vi "check_instrument_error.vi"(6 "Mode (Check error from Session)":T1(ring)=enum."Check error from Session", 7 "Attribute":T2={"Identifier"="", "Descriptive Name"="", "Data Type"=enum."Integer 32", "Command"="", "Access"=enum."Read/Write", "Range Table"="", "Read Callback"="", "Write Callback"="", "Supported Models"="", "Instrument Options"="", "Index"=0, "OPC Wait"=FALSE, "No Status Check"=FALSE, "Cache Only"=FALSE}, 8 "error in":errorcluster caption="error in (no error)", 11 "VISA resource name":refnum<visa-resource-name>) -> (0 "error out":errorcluster, 3 "VISA resource name out":refnum<visa-resource-name>)   [LabVIEW 2020, in "Rohde&Schwarz RTx Oscilloscopes.lvlib" / "rsidr_core.lvlib"]
uses:
  rsidr_core.lvlib
  type_Attribute.ctl
  type_Attribute_Data_Type.ctl
  type_ReadWriteAccess.ctl
  type_AdditionalFlag_Bits.ctl
  type_Error_Codes.ctl
  Match Regular Expression.xnode
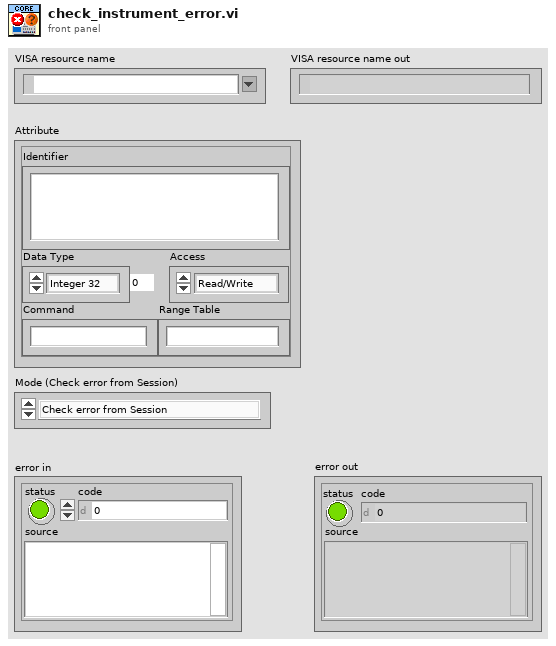
[diagram p1: front panel]
types:
  T1 = enum16{"Check error", "Don't check error", "Check error from Session"}
  T2 = typedef "Rohde&Schwarz RTx Oscilloscopes.lvlib/rsidr_core.lvlib/type_Attribute.ctl" = cluster{"Identifier":string, "Descriptive Name":string, "Data Type":T3, "Command":string, "Access":T4, "Range Table":string, "Read Callback":string, "Write Callback":string, "Supported Models":string, "Instrument Options":string, "Index":i32, "OPC Wait":bool, "No Status Check":bool, "Cache Only":bool}
  T3 = typedef "Rohde&Schwarz RTx Oscilloscopes.lvlib/rsidr_core.lvlib/type_Attribute_Data_Type.ctl" = enum16{"Integer 32", "Double", "String", "Boolean", "None", "Integer 64", "RawString"}
  T4 = typedef "Rohde&Schwarz RTx Oscilloscopes.lvlib/rsidr_core.lvlib/type_ReadWriteAccess.ctl" = enum16{"Read Only", "Write Only", "Read/Write"}
  T5 = typedef "Rohde&Schwarz RTx Oscilloscopes.lvlib/rsidr_core.lvlib/type_AdditionalFlag_Bits.ctl" = enum16{"Send LF after Bin Block", "Junk read with io_clear_buffers.vi", "io_clear_buffers: viClear()", "io_clear_buffers: viFlush()", "<NotUsed1>", "Allow Dbl & Int Bin/Ascii read", "*OPC? in check_instrument_error.vi", "<NotUsed2>", "Smart Enum Matching", "Less Strict RepCaps check", "AssureResponseEndWithLF"}
  T6 = typedef "Rohde&Schwarz RTx Oscilloscopes.lvlib/rsidr_core.lvlib/type_Session_Data.ctl" = cluster{"IDN string":string, "Instrument FW":string, "Instr type":string, "Instr type for err. msg.":string, "Installed Options":string[], "Ignore Error Messages":string, "Logging params":variant, "OPC Timeout":i32, "VISA Timeout":i32, "STB Poll VISA Timeout":i32, "Additional Flags":i32, "Wait Before Read":i32, "Wait Before Write":i32, "Option String Flags":i32, "IO Segment Size":i64, "VISA Access Mode":T7, "Interface Type":T8, "OPC Wait Mode":T9, "Bin Float Number  Format":T10, "Bin Integer Number Format":T11, "Simulate":bool, "VXIcapable":bool, "Duplicate Session":bool, "Add LF to Write":bool, "Logging":bool, "Fast Sweep":bool, "Query Instrument Status":bool, "Check Range":bool, "Check Options":bool, "OPC-sync Attr Writes":bool, "OPC-sync Attr Queries":bool}
  T7 = typedef "Rohde&Schwarz RTx Oscilloscopes.lvlib/rsidr_core.lvlib/type_VisaAccessMode.ctl" = u16
  T8 = typedef "Rohde&Schwarz RTx Oscilloscopes.lvlib/rsidr_core.lvlib/type_InterfaceType.ctl" = enum16{"Unknown", "GPIB", "VXI", "GPIB_VXI", "ASRL", "PXI", "TCPIP", "USB", "SOCKET"}
  T9 = typedef "Rohde&Schwarz RTx Oscilloscopes.lvlib/rsidr_core.lvlib/type_OPC_Wait_Mode.ctl" = enum16{"STBpolling", "STBpollingSlow", "STBpollingSuperSlow", "ServiceRequest", "OPCquery"}
  T10 = typedef "Rohde&Schwarz RTx Oscilloscopes.lvlib/rsidr_core.lvlib/type_Binary_Float_Number_Format.ctl" = enum16{"Float_4_Bytes_Swapped", "Float_4_Bytes", "Double_8_Bytes_Swapped", "Double_8_Bytes"}
  T11 = typedef "Rohde&Schwarz RTx Oscilloscopes.lvlib/rsidr_core.lvlib/type_Binary_Integer_Number_Format.ctl" = enum16{"Int32_4_Bytes_Swapped", "Int32_4 Bytes", "Int16_2_Bytes_Swapped", "Int16_2_Bytes"}
  T12 = typedef "Rohde&Schwarz RTx Oscilloscopes.lvlib/rsidr_core.lvlib/type_Error_Codes.ctl" = enum16{"No_error", "VISA_err_ResourceNotFound", "VISA_err_Timeout", "VISA_warn_MoreDataAvailable", "RS_err_MissingCallback", "RS_err_InvalidAttribute", "RS_err_InvalidValue", "RS_err_UnknownResource", "RS_err_AlreadyInitialized", "RS_err_InstrumentStatus", "RS_err_BadRepCapName", "RS_err_TypesMismatch", "RS_err_ValueNotSupported", "RS_err_InvalidRngTable", "RS_err_IDqueryFail", "RS_err_UnexpResponse", "VISA_warn_ConfigNotLoaded", "RS_err_AttributeNotReadable", "RS_err_AttributeNotWritable", "RS_err_InstrumentType", "RS_err_InstrumentOption", "VISA_err_InvalidSize", "RS_err_ReliabilityIndicator", "VISA_warn_UnknownStatus", "VISA_warn_TermCharRead", "VISA_err_IO_error", "RS_err_FunctionNotSupported", "VISA_warn_QueueEmpty"}
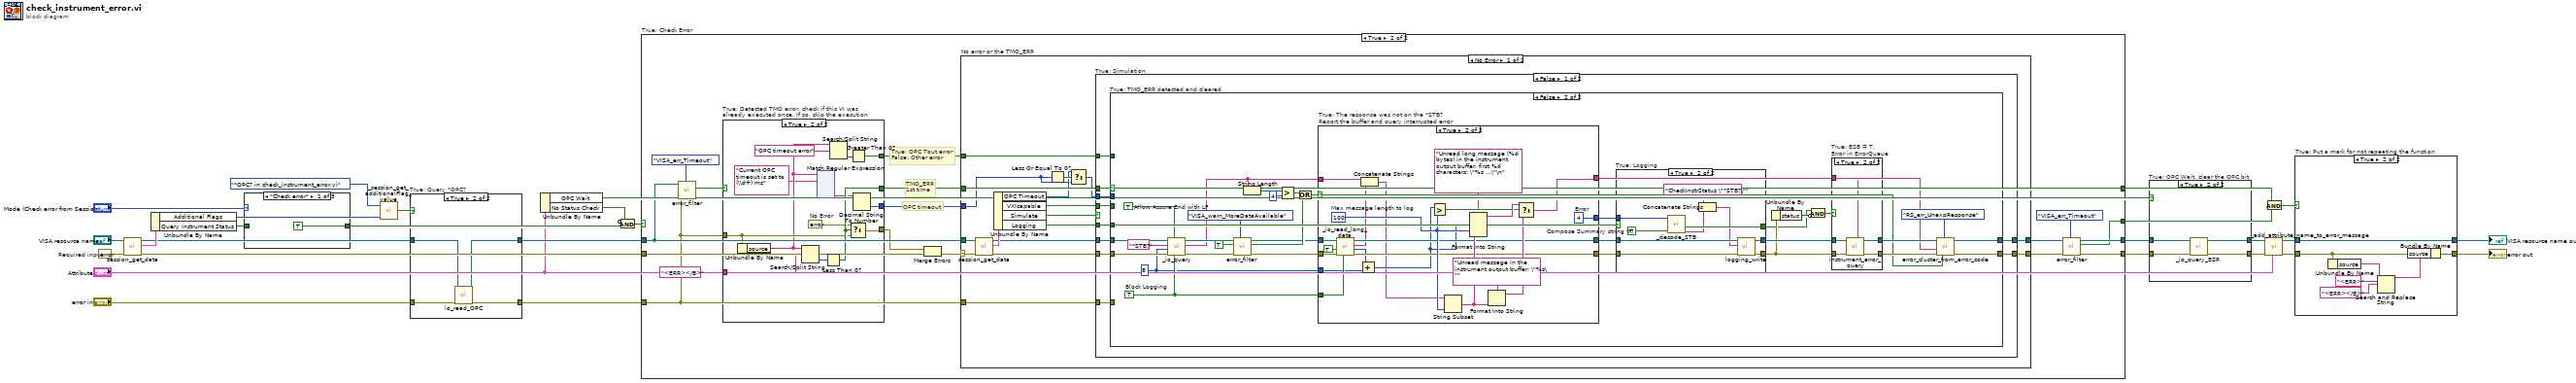
[diagram p0: block diagram]
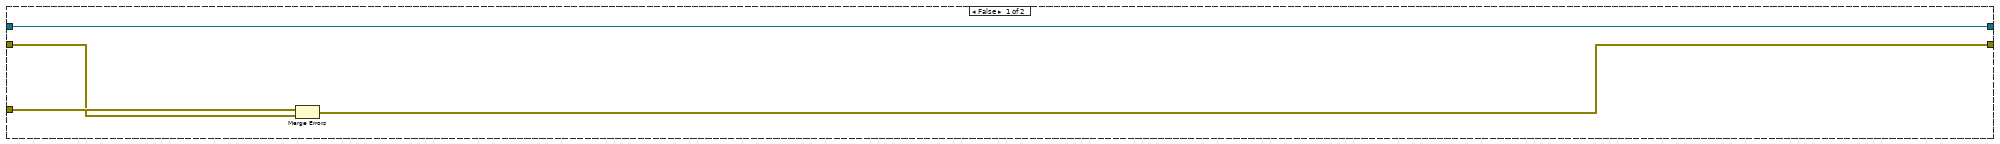
[diagram p5: hidden frame]
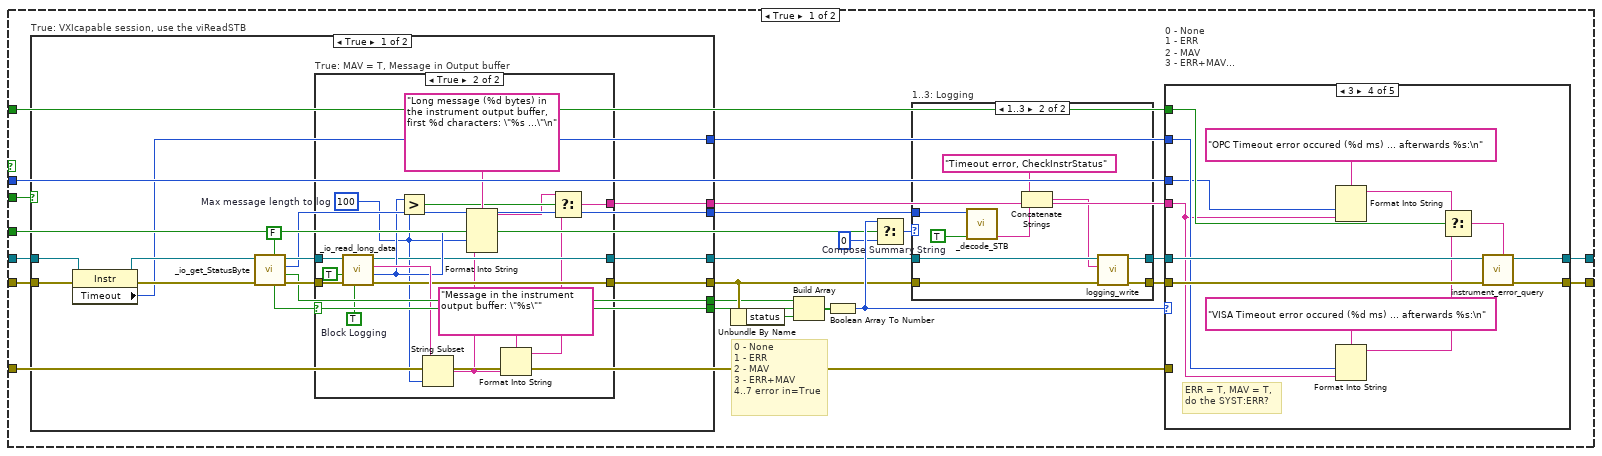
[diagram p7: hidden frame]
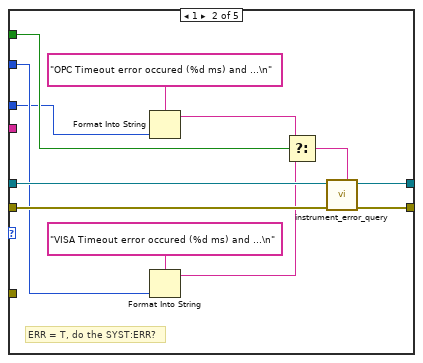
[diagram p9: hidden frame]
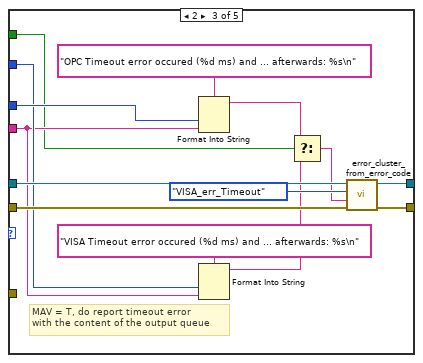
[diagram p10: hidden frame]
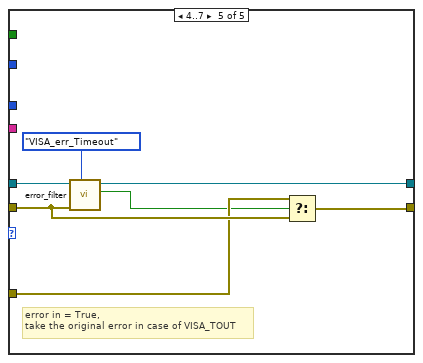
[diagram p11: hidden frame]
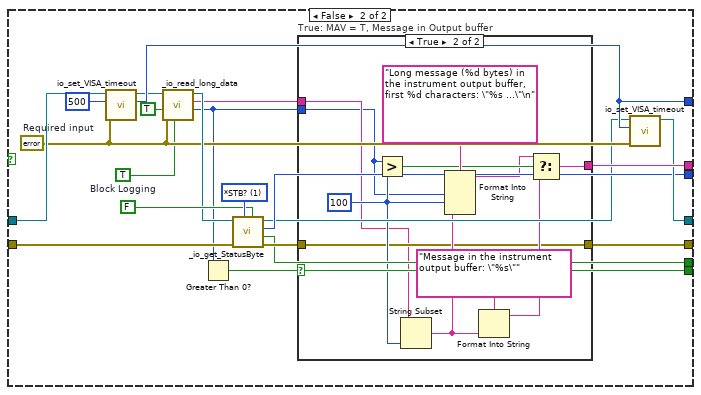
[diagram p14: hidden frame]
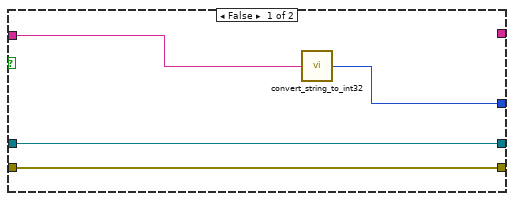
[diagram p16: hidden frame]
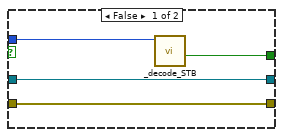
[diagram p18: hidden frame]
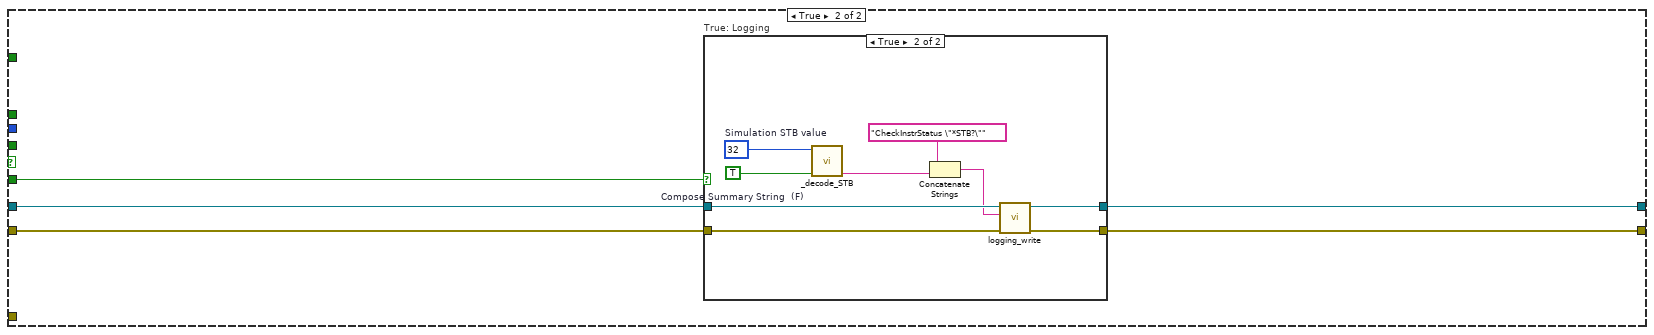
[diagram p19: hidden frame]
diagram:
  w20 = errorcluster {"status"=FALSE, "code"=0, "source"=""}  # Required input
  n1 = call "session_get_data.vi"("error in"=w20, "VISA resource name"="VISA resource name") -> ("error out"=w16:errorcluster, "Session User Data out"=w21:T6, "VISA resource name out"=w18:refnum<visa-resource-name>)  [unwired: 6 in, 1 out]
  n2 = Unbundle By Name(w21) -> ("Additional Flags"=w4:i32, "Query Instrument Status"=w19:bool)
  n3 = case shown="\"Check error\"" "Mode (Check error from Session)" {
    tunnel: [TRUE ("Boolean Out") _ w31] -> w28
    tunnel: w19 -> [_ _ w31]
    frame "Check error" {
    }
    frame "Don't check error" {
    }
    frame "Check error from Session" {
    }
  }
  n4 = call "_session_get_additionalFlag_value.vi"("AdditionalFlags value in"=w4, "AdditionalFlag bit"=type_AdditionalFlag_Bits."*OPC? in check_instrument_error.vi") -> ("AdditionalFlag bit value out"=w5:bool)  [unwired: 3 in]
  n5 = case "True: Query *OPC?" shown="True" w5 {
    tunnel: w18 -> [w32 w35]
    tunnel: [w32 w34] -> w17
    tunnel: "error in" -> [w33 w37]
    tunnel: [w33 w36] -> w14
    frame False {
    }
    frame True {
      n6 = call "io_read_OPC.vi"("error in"=w37, "VISA resource name"=w35) -> ("error out"=w36:errorcluster, "VISA resource name out"=w34:refnum<visa-resource-name>)  [unwired: 7 in, 1 out]
    }
  }
  n7 = Unbundle By Name("Attribute") -> ("OPC Wait"=w26:bool, "No Status Check"=w23:bool)
  n8 = Compound Arithmetic op=AND(invert w23, w28) -> (w27:bool)
  n9 = case "True: Check Error" shown="True" w27 {
    tunnel: [w41 w45] -> w24
    tunnel: [w39 w46] -> w25
    tunnel: w17 -> [w41 w56]
    tunnel: w16 -> [w38 w57]
    tunnel: w14 -> [w40 w53]
    tunnel: [_ w50] -> w7
    tunnel: [_ w44] -> w6
    frame False {
      n10 = Merge Errors(w40, w38) -> (w39:errorcluster)
    }
    frame True {
      # "OPC timeout"
      # "True: OPC Tout error\nFalse: Other error"
      # "TMO_ERR\n1st time"
      n11 = call "error_filter.vi"("Error Enum in"=type_Error_Codes."VISA_err_Timeout", "error in"=w53, "VISA resource name"=w56) -> ("Code Detected"=w54:bool)  [unwired: 6 in, 2 out]
      n12 = case "True: Detected TMO error, check if this VI was\nalready executed once. If so, skip the execution" shown="True" w54 {
        tunnel: w53 -> [w59 w69]
        tunnel: [w59 w71] -> w52
        tunnel: [_ w70] -> w50
        tunnel: "<ERR></B>" ("search string/char (-)") -> [_ w67]
        tunnel: [_ w65] -> w43
        tunnel: [_ w61] -> w42
        frame False {
        }
        frame True {
          w68 = errorcluster {"status"=FALSE, "code"=0, "source"=""}  # No Error
          n13 = Unbundle By Name(w69) -> ("source"=w63:string)
          n14 = Search/Split String(string=w63, search string/char (-)=w67) -> (offset of match=w72:i32)  [unwired: 1 in, 2 out]
          n15 = xnode "Match Regular Expression"("input string"=w63, "regular expression"="Current OPC timeout is set to (\\d+) ms") -> ("submatch 1"=w62:string)  [unwired: 4 in, 5 out]
          n16 = Less Than 0?(x=w72) -> (x < 0?=w70:bool)
          n17 = Search/Split String(string=w63, search string/char (-)="OPC timeout error") -> (offset of match=w66:i32)  [unwired: 1 in, 2 out]
          n18 = Select(t=w68, s=w70, f=w69) -> (s? t:f=w71:errorcluster)
          n19 = Greater Than 0?(x=w66) -> (x > 0?=w65:bool)
          n20 = Decimal String To Number(string=w62) -> (number=w61:i32)  [unwired: 2 in, 1 out]
        }
      }
      n21 = Merge Errors(w52, w57) -> (w55:errorcluster)
      n22 = case "No error or the TMO_ERR" shown="No Error" w55 {
        selector: w55 -> [w196 w455]
        tunnel: [w201 w456] -> w47
        tunnel: [w202 w455] -> w48
        tunnel: w56 -> [w200 w456]
        tunnel: w50 -> [w195 _]
        tunnel: w53 -> [w194 _]
        tunnel: w43 -> [w191 _]
        tunnel: w42 -> [w187 _]
        frame No Error {
          n23 = call "session_get_data.vi"("error in"=w196, "VISA resource name"=w200) -> ("error out"=w198:errorcluster, "Session User Data out"=w199:T6, "VISA resource name out"=w197:refnum<visa-resource-name>)  [unwired: 6 in, 1 out]
          n24 = Unbundle By Name(w199) -> ("OPC Timeout"=w188:i32, "VXIcapable"=w190:bool, "Simulate"=w193:bool, "Logging"=w192:bool)
          n25 = Less Or Equal To 0?(x=w187) -> (x <= 0?=w189:bool)
          n26 = Select(t=w188, s=w189, f=w187) -> (s? t:f=w186:i32)
          n27 = case "True: Simulation" shown="False" w193 {
            tunnel: [w207 w441] -> w202
            tunnel: [w208 w440] -> w201
            tunnel: w198 -> [w211 w443]
            tunnel: w197 -> [w212 w442]
            tunnel: w195 -> [w210 _]
            tunnel: w190 -> [w209 _]
            tunnel: w194 -> [w206 _]
            tunnel: w192 -> [w205 w439]
            tunnel: w186 -> [w204 _]
            tunnel: w191 -> [w203 _]
            frame False {
              n28 = case "True: TMO_ERR detected and cleared" shown="False" w210 {
                tunnel: w212 -> [w222 w391]
                tunnel: w211 -> [w221 w390]
                tunnel: [w218 w364] -> w208
                tunnel: [w217 w365] -> w207
                tunnel: w209 -> [w220 _]
                tunnel: w206 -> [w215 _]
                tunnel: w205 -> [w216 w383]
                tunnel: w204 -> [w214 _]
                tunnel: w203 -> [w213 _]
                frame True {
                  # "0 - None\n1 - ERR\n2 - MAV\n3 - ERR+MAV\n4..7 error in=True"
                  n29 = case "True: VXIcapable session, use the viReadSTB" shown="True" w220 {
                    tunnel: w222 -> [w298 w346]
                    tunnel: w221 -> [w300 w343]
                    tunnel: [w306 w342] -> w229
                    tunnel: [w304 w332] -> w227
                    tunnel: [w305 w341] -> w226
                    tunnel: [w303 w340] -> w232
                    tunnel: [w302 w339] -> w230
                    tunnel: [w301 w338] -> w231
                    tunnel: [w296 w337] -> w219
                    frame True {
                      n30 = property on="Property Node" class="Instr"(reference=w298, error in=w300) -> (reference out=w297:refnum<visa-resource-name>, error out=w299:errorcluster, "Timeout"=w296:u32)
                      n31 = call "_io_get_StatusByte.vi"("Block Setting of VISA Timeout for viReadSTB"=FALSE, "error in"=w299, "VISA resource name"=w297) -> ("error out"=w307:errorcluster, "Error"=w305:bool, "STB returned"=w301:u16, "VISA resource name out"=w308:refnum<visa-resource-name>, "MAV"=w304:bool)  [unwired: 3 in, 1 out]
                      n32 = case "True: MAV = T, Message in Output buffer" shown="True" w304 {
                        tunnel: w307 -> [w310 w326]
                        tunnel: w308 -> [w309 w324]
                        tunnel: [w310 w320] -> w306
                        tunnel: [w309 w321] -> w302
                        tunnel: [_ w313] -> w303
                        frame False {
                        }
                        frame True {
                          w312 = u32 100  # Max message length to log
                          w325 = TRUE  # Block Logging
                          n33 = call "_io_read_long_data.vi"("Block Logging (F)"=w325, "error in"=w326, "Trim Response End (T)"=TRUE, "VISA resource name"=w324) -> ("error out"=w320:errorcluster, "Read bytes count"=w322:u32, "Read buffer"=w323:string, "VISA resource name out"=w321:refnum<visa-resource-name>)  [unwired: 4 in]
                          n34 = Greater?(x=w322, y=w312) -> (0:w316:bool)
                          n35 = String Subset(string=w323, length (rest)=w312) -> (substring=w318:string)  [unwired: 1 in]
                          n36 = Format Into String(format string="Long message (%d bytes) in the instrument output buffer, first %d characters: \"%s ...\"\n", w322, w312, w318) -> (resulting string=w315:string)  [unwired: 2 in, 1 out]
                          n37 = Format Into String(format string="Message in the instrument output buffer: \"%s\"", w318) -> (resulting string=w314:string)  [unwired: 2 in, 1 out]
                          n38 = Select(t=w315, s=w316, f=w314) -> (s? t:f=w313:string)
                        }
                      }
                    }
                    frame False {
                      w328 = TRUE  # Block Logging
                      w333 = errorcluster {"status"=FALSE, "code"=0, "source"=""}  # Required input
                      w344 = u16 1 items=["viReadSTB", "*STB?"] ("Method (viReadSTB)")
                      n39 = call "io_set_VISA_timeout.vi"("error in"=w333, "VISA Timeout"=u32 500, "VISA resource name"=w346) -> ("Old VISA Timeout"=w337:u32, "VISA resource name out"=w335:refnum<visa-resource-name>)  [unwired: 6 in, 1 out]
                      n40 = call "_io_read_long_data.vi"("Block Logging (F)"=w328, "error in"=w333, "Trim Response End (T)"=TRUE, "VISA resource name"=w335) -> ("Read bytes count"=w330:u32, "Read buffer"=w331:string, "VISA resource name out"=w334:refnum<visa-resource-name>)  [unwired: 4 in, 1 out]
                      n41 = Greater Than 0?(x=w330) -> (x > 0?=w332:bool)
                      n42 = call "_io_get_StatusByte.vi"("Block Setting of VISA Timeout for viReadSTB"=FALSE, "Method (viReadSTB)"=w344, "error in"=w343, "VISA resource name"=w334) -> ("error out"=w347:errorcluster, "Error"=w341:bool, "STB returned"=w338:u16, "VISA resource name out"=w329:refnum<visa-resource-name>)  [unwired: 2 in, 2 out]
                      n43 = case "True: MAV = T, Message in Output buffer" shown="True" w332 {
                        tunnel: w347 -> [w348 w351]
                        tunnel: [w348 w351] -> w342
                        tunnel: [_ w352] -> w340
                        tunnel: w331 -> [_ w350]
                        tunnel: w330 -> [_ w349]
                        frame False {
                        }
                        frame True {
                          w359 = u32 100 ("y")
                          n44 = Greater?(x=w349, y=w359) -> (0:w355:bool)
                          n45 = String Subset(string=w350, length (rest)=w359) -> (substring=w357:string)  [unwired: 1 in]
                          n46 = Format Into String(format string="Long message (%d bytes) in the instrument output buffer, first %d characters: \"%s ...\"\n", w349, w359, w357) -> (resulting string=w354:string)  [unwired: 2 in, 1 out]
                          n47 = Format Into String(format string="Message in the instrument output buffer: \"%s\"", w357) -> (resulting string=w353:string)  [unwired: 2 in, 1 out]
                          n48 = Select(t=w354, s=w355, f=w353) -> (s? t:f=w352:string)
                        }
                      }
                      n49 = call "io_set_VISA_timeout.vi"("error in"=w333, "VISA Timeout"=w337, "VISA resource name"=w329) -> ("VISA resource name out"=w339:refnum<visa-resource-name>)  [unwired: 6 in, 2 out]
                    }
                  }
                  n50 = Unbundle By Name(w229) -> ("status"=w225:bool)
                  n51 = Build Array(w226, w227, w225) -> (w224:bool[])
                  n52 = Boolean Array To Number(Boolean array=w224) -> (number=w235:u32)
                  n53 = Select(t=w235, s=w216, f=u32 0) -> (s? t:f=w228:u32)
                  n54 = case "1..3: Logging" shown="1..3" w228 {
                    tunnel: w229 -> [w285 w293]
                    tunnel: [w285 w292] -> w234
                    tunnel: [w284 w291] -> w233
                    tunnel: w230 -> [w284 w290]
                    tunnel: w231 -> [_ w287]
                    frame Default {
                    }
                    frame 1..3 {
                      w294 = TRUE  # Compose Summary String
                      n55 = call "_decode_STB.vi"("Compose Summary string (F)"=w294, "STB in"=w287) -> ("Summary string"=w286:string)  [unwired: 6 in, 3 out]
                      n56 = Concatenate Strings("Timeout error, CheckInstrStatus" ("String to write"), w286) -> (w288:string)
                      n57 = call "logging_write.vi"("error in"=w293, "String to write"=w288, "VISA resource name"=w290) -> ("error out"=w292:errorcluster, "VISA resource name out"=w291:refnum<visa-resource-name>)  [unwired: 7 in]
                    }
                  }
                  n58 = case "0 - None\n1 - ERR\n2 - MAV\n3 - ERR+MAV\n4..7 error in=True" shown="3" w235 {
                    tunnel: w215 -> [w236 _ _ _ w278]
                    tunnel: [w236 w249 w259 w276 w280] -> w217
                    tunnel: w233 -> [w237 w246 w261 w273 w282]
                    tunnel: [w237 w248 w263 w275 w281] -> w218
                    tunnel: w234 -> [_ w245 w260 w272 w279]
                    tunnel: w232 -> [_ _ w254 w264 _]
                    tunnel: w219 -> [_ w244 w255 w271 _]
                    tunnel: w214 -> [_ w241 w257 w268 _]
                    tunnel: w213 -> [_ w243 w251 w270 _]
                    frame 0, Default {
                      # "ERR = F, MAV = F, pass the TMO_ERR forward"
                    }
                    frame 1 {
                      # "ERR = T, do the SYST:ERR?"
                      n59 = Format Into String(format string="OPC Timeout error occured (%d ms) and ...\n" ("Beginning error message string (\"\")"), w241) -> (resulting string=w240:string)  [unwired: 2 in, 1 out]
                      n60 = Format Into String(format string="VISA Timeout error occured (%d ms) and ...\n" ("Beginning error message string (\"\")"), w244) -> (resulting string=w239:string)  [unwired: 2 in, 1 out]
                      n61 = Select(t=w240, s=w243, f=w239) -> (s? t:f=w238:string)
                      n62 = call "instrument_error_query.vi"("Beginning error message string (\"\")"=w238, "error in"=w245, "VISA resource name"=w246) -> ("error out"=w249:errorcluster, "VISA resource name out"=w248:refnum<visa-resource-name>)  [unwired: 5 in, 2 out]
                    }
                    frame 2 {
                      # "MAV = T, do report timeout error\nwith the content of the output queue"
                      n63 = Format Into String(format string="OPC Timeout error occured (%d ms) and ... afterwards: %s\n" ("Beginning error message string (\"\")"), w257, w254) -> (resulting string=w253:string)  [unwired: 2 in, 1 out]
                      n64 = Format Into String(format string="VISA Timeout error occured (%d ms) and ... afterwards: %s\n" ("Beginning error message string (\"\")"), w255, w254) -> (resulting string=w252:string)  [unwired: 2 in, 1 out]
                      n65 = Select(t=w253, s=w251, f=w252) -> (s? t:f=w250:string)
                      n66 = call "error_cluster_from_error_code.vi"("error in"=w260, "Error Message (\"\")"=w250, "Error Enum in"=type_Error_Codes."VISA_err_Timeout", "VISA resource name"=w261) -> ("error out"=w259:errorcluster, "VISA resource name out"=w263:refnum<visa-resource-name>)  [unwired: 6 in]
                    }
                    frame 3 {
                      # "ERR = T, MAV = T,\ndo the SYST:ERR?"
                      n67 = Format Into String(format string="OPC Timeout error occured (%d ms) ... afterwards %s:\n" ("Beginning error message string (\"\")"), w268, w264) -> (resulting string=w267:string)  [unwired: 2 in, 1 out]
                      n68 = Format Into String(format string="VISA Timeout error occured (%d ms) ... afterwards %s:\n" ("Beginning error message string (\"\")"), w271, w264) -> (resulting string=w266:string)  [unwired: 2 in, 1 out]
                      n69 = Select(t=w267, s=w270, f=w266) -> (s? t:f=w265:string)
                      n70 = call "instrument_error_query.vi"("Beginning error message string (\"\")"=w265, "error in"=w272, "VISA resource name"=w273) -> ("error out"=w276:errorcluster, "VISA resource name out"=w275:refnum<visa-resource-name>)  [unwired: 5 in, 2 out]
                    }
                    frame 4..7 {
                      # "error in = True,\ntake the original error in case of VISA_TOUT"
                      n71 = call "error_filter.vi"("Error Enum in"=type_Error_Codes."VISA_err_Timeout", "error in"=w279, "VISA resource name"=w282) -> ("Code Detected"=w277:bool, "VISA resource name out"=w281:refnum<visa-resource-name>)  [unwired: 6 in, 1 out]
                      n72 = Select(t=w278, s=w277, f=w279) -> (s? t:f=w280:errorcluster)
                    }
                  }
                }
                frame False {
                  w360 = TRUE  # Allow Assure End with LF
                  w369 = TRUE  # Block Logging
                  w368 = u32 8 ("byte count (0)")
                  n73 = call "_io_query.vi"("Block Logging (F)"=w369, "Allow Assure End with LF"=w360, "error in"=w390, "Max bytes to read (2048)"=w368, "Write buffer"="*STB?" ("write buffer (\"\")"), "VISA resource name"=w391) -> ("error out"=w378:errorcluster, "Read buffer"=w376:string, "VISA resource name out"=w377:refnum<visa-resource-name>)  [unwired: 2 in, 1 out]
                  n74 = call "error_filter.vi"("Error Enum in"=type_Error_Codes."VISA_warn_MoreDataAvailable", "error in"=w378, "Clear detected code (F)"=TRUE, "VISA resource name"=w377) -> ("error out"=w372:errorcluster, "Code Detected"=w374:bool, "VISA resource name out"=w373:refnum<visa-resource-name>)  [unwired: 5 in]
                  n75 = String Length(string=w376) -> (length=w382:i32)
                  n76 = Greater?(x=w382, y=4) -> (0:w375:bool)
                  n77 = Or(x=w375, y=w374) -> (x .or. y?=w361:bool)
                  n78 = case "True: The response was not on the *STB?\nReport the buffer and query interrupted error" shown="True" w361 {
                    tunnel: [w393 w417] -> w389
                    tunnel: w376 -> [w396 w400]
                    tunnel: [_ w405] -> w363
                    tunnel: w373 -> [w394 w409]
                    tunnel: w372 -> [w395 w408]
                    tunnel: [w394 w407] -> w371
                    tunnel: [w395 w406] -> w370
                    tunnel: w369 -> [_ w404]
                    tunnel: w368 -> [_ w403]
                    frame False {
                      n79 = call "convert_string_to_int32.vi"("String in"=w396) -> ("int32 value out"=w393:i32)  [unwired: 4 in]
                    }
                    frame True {
                      w416 = u32 100  # Max message length to log
                      w417 = 4  # Error
                      n80 = call "_io_read_long_data.vi"("Block Logging (F)"=w404, "error in"=w408, "Trim Response End (T)"=TRUE, "VISA resource name"=w409) -> ("error out"=w406:errorcluster, "Read bytes count"=w402:u32, "Read buffer"=w399:string, "VISA resource name out"=w407:refnum<visa-resource-name>)  [unwired: 4 in]
                      n81 = Add(x=w402, y=w403) -> (x+y=w401:u32)
                      n82 = Concatenate Strings(w400, w399) -> (w398:string)
                      n83 = Greater?(x=w401, y=w416) -> (0:w413:bool)
                      n84 = String Subset(string=w398, length (rest)=w416) -> (substring=w411:string)  [unwired: 1 in]
                      n85 = Format Into String(format string="Unread long message (%d bytes) in the instrument output buffer, first %d characters: \"%s ...\"\n", w401, w416, w411) -> (resulting string=w414:string)  [unwired: 2 in, 1 out]
                      n86 = Format Into String(format string="Unread message in the instrument output buffer: \"%s\"", w411) -> (resulting string=w415:string)  [unwired: 2 in, 1 out]
                      n87 = Select(t=w414, s=w413, f=w415) -> (s? t:f=w405:string)
                    }
                  }
                  n88 = case "True: Logging" shown="True" w383 {
                    tunnel: w370 -> [w427 w438]
                    tunnel: [w427 w437] -> w387
                    tunnel: [w426 w436] -> w388
                    tunnel: w371 -> [w426 w435]
                    tunnel: [w428 w434] -> w385
                    tunnel: w389 -> [w425 w431]
                    frame False {
                      n89 = call "_decode_STB.vi"("STB in"=w425) -> ("Error"=w428:bool)  [unwired: 7 in, 3 out]
                    }
                    frame True {
                      w429 = TRUE  # Compose Summary string (F)
                      n90 = call "_decode_STB.vi"("Compose Summary string (F)"=w429, "STB in"=w431) -> ("Summary string"=w430:string, "Error"=w434:bool)  [unwired: 6 in, 2 out]
                      n91 = Concatenate Strings("CheckInstrStatus \"*STB?\"" ("String to write"), w430) -> (w432:string)
                      n92 = call "logging_write.vi"("error in"=w438, "String to write"=w432, "VISA resource name"=w435) -> ("error out"=w437:errorcluster, "VISA resource name out"=w436:refnum<visa-resource-name>)  [unwired: 7 in]
                    }
                  }
                  n93 = Unbundle By Name(w387) -> ("status"=w386:bool)
                  n94 = Compound Arithmetic op=AND(w385, invert w386) -> (w384:bool)
                  n95 = case "True: ESB = T,\nError in ErrorQueue" shown="True" w384 {
                    tunnel: [w418 w424] -> w367
                    tunnel: [w419 w423] -> w366
                    tunnel: w387 -> [w418 w422]
                    tunnel: w388 -> [w419 w421]
                    tunnel: w363 -> [_ w420]
                    frame False {
                    }
                    frame True {
                      n96 = call "instrument_error_query.vi"("Beginning error message string (\"\")"=w420, "error in"=w422, "VISA resource name"=w421) -> ("error out"=w424:errorcluster, "VISA resource name out"=w423:refnum<visa-resource-name>)  [unwired: 5 in, 2 out]
                    }
                  }
                  n97 = call "error_cluster_from_error_code.vi"("Error Creation Enabled (True)"=w361, "error in"=w367, "Error Message (\"\")"=w363, "Error Enum in"=type_Error_Codes."RS_err_UnexpResponse", "VISA resource name"=w366) -> ("error out"=w365:errorcluster, "VISA resource name out"=w364:refnum<visa-resource-name>)  [unwired: 5 in]
                }
              }
            }
            frame True {
              n98 = case "True: Logging" shown="True" w439 {
                tunnel: w443 -> [w445 w454]
                tunnel: w442 -> [w444 w453]
                tunnel: [w445 w452] -> w441
                tunnel: [w444 w451] -> w440
                frame False {
                }
                frame True {
                  w449 = TRUE  # Compose Summary String  (F)
                  w450 = u16 32  # Simulation STB value
                  n99 = call "_decode_STB.vi"("Compose Summary string (F)"=w449, "STB in"=w450) -> ("Summary string"=w446:string)  [unwired: 6 in, 3 out]
                  n100 = Concatenate Strings("CheckInstrStatus \"*STB?\"" ("String to write"), w446) -> (w447:string)
                  n101 = call "logging_write.vi"("error in"=w454, "String to write"=w447, "VISA resource name"=w453) -> ("error out"=w452:errorcluster, "VISA resource name out"=w451:refnum<visa-resource-name>)  [unwired: 7 in]
                }
              }
            }
          }
        }
        frame Error {
          # "Communication error or error\nchecking turned off"
        }
      }
      n102 = call "error_filter.vi"("Error Enum in"=type_Error_Codes."VISA_err_Timeout", "error in"=w48, "VISA resource name"=w47) -> ("error out"=w46:errorcluster, "Code Detected"=w44:bool, "VISA resource name out"=w45:refnum<visa-resource-name>)  [unwired: 6 in]
    }
  }
  n103 = case "True: OPC Wait, clear the OPC bit" shown="True" w26 {
    tunnel: w25 -> [w458 w462]
    tunnel: w24 -> [w457 w461]
    tunnel: [w458 w460] -> w11
    tunnel: [w457 w459] -> w2
    frame False {
    }
    frame True {
      n104 = call "_io_query_ESR.vi"("error in"=w462, "VISA resource name"=w461) -> ("error out"=w460:errorcluster, "VISA resource name out"=w459:refnum<visa-resource-name>)  [unwired: 7 in, 1 out]
    }
  }
  n105 = call "_add_attribute_name_to_error_message.vi"("Attribute"="Attribute", "error in"=w11, "VISA resource name"=w2) -> ("error out"=w10:errorcluster, "VISA resource name out"=w1:refnum<visa-resource-name>)  [unwired: 6 in, 1 out]
  n106 = And(x=w7, y=w6) -> (x .and. y?=w9:bool)
  n107 = case "True: Put a mark for not repeating the function" shown="True" w9 {
    tunnel: w10 -> [w464 w466]
    tunnel: w1 -> [w463 w468]
    tunnel: [w463 w468] -> w13
    tunnel: [w464 w467] -> w12
    frame False {
    }
    frame True {
      n108 = Unbundle By Name(w466) -> ("source"=w470:string)
      n109 = Search and Replace String(input string=w470, search string="<ERR>", replace string="<ERR></B>" ("replace string (\"\")")) -> (result string=w465:string)  [unwired: 5 in, 3 out]
      n110 = Bundle By Name(cluster=w466, "source"=w465) -> (w467:errorcluster)
    }
  }
  "error out" <- w12
  "VISA resource name out" <- w13
